vi "Finish.vi"(6 "Sender":refnum<class "Sender.lvclass">, 9 "Error":errorcluster, 10 "Actor":refnum<class "Actor.lvclass">) -> (2 "Msg":refnum<class "Msg.lvclass">)   [LabVIEW 2025, in "jettl.lvlib" / "Finish Msg.lvlib"]
uses:
  Finish Msg.lvlib
  Msg/Msg.lvclass
  Actor/Actor/Actor.lvclass
  Sender/Sender/Sender.lvclass
  Finish Msg/Finish Msg.lvclass
  C:/git/jettl/src/jettl/jettl/Msg/Msg.lvclass
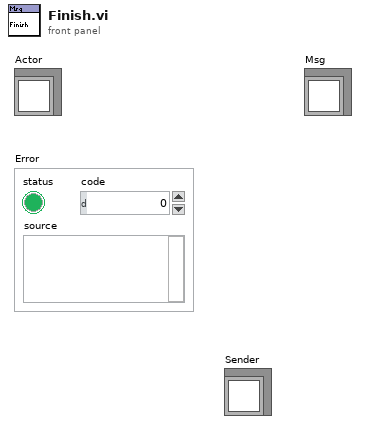
[diagram p1: front panel]
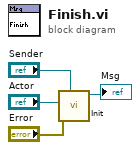
[diagram p0: block diagram]
diagram:
  n1 = call "Init.vi"("Sender"="Sender", "Error"="Error", "Actor"="Actor") -> ("Finish Msg out"=→"Msg":refnum<class "Finish Msg.lvclass">)  [unwired: 8 in]
